vi "Clear Controls.vi"(8 "error in (no error)":errorcluster, 10 "Array 2":refnum<vi>[](array[refnum]), 11 "Array":refnum<vi>[](array[refnum])) -> (0 "error out":errorcluster)   [LabVIEW 2020]
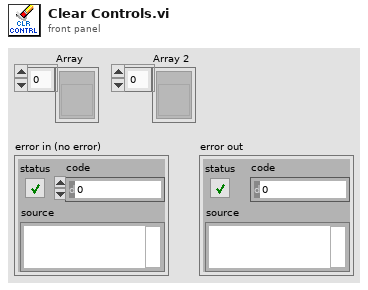
[diagram p1: front panel]
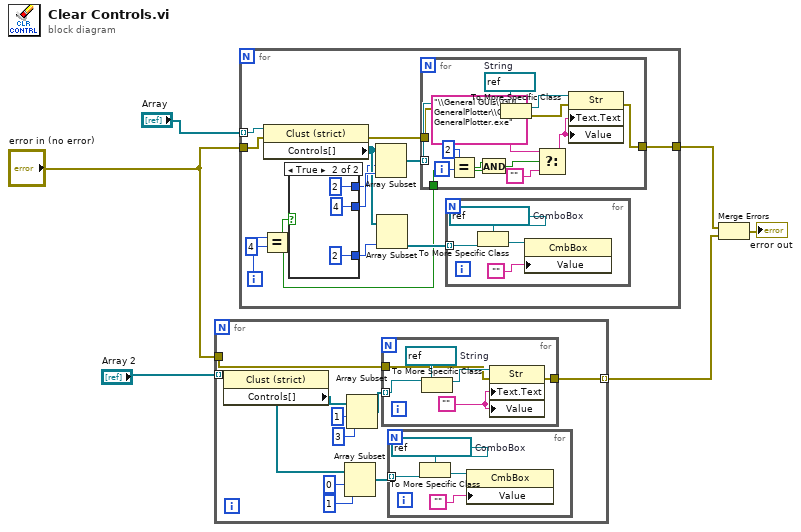
[diagram p0: block diagram]
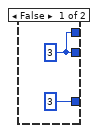
[diagram p2: hidden frame]
diagram:
  n1 = for {
    tunnel: "Array 2" -> [w13] mode=indexing
    tunnel: "error in (no error)" -> [w12]
    tunnel: [w7] -> w3 mode=indexing
    n2 = property class="Clust (strict)"(reference=w13) -> ("Controls[]"=w11:refnum<vi>[])  [unwired: 1 in, 2 out]
    n3 = Array Subset(array=w11, index=0, length=1) -> (w8:refnum<vi>[])
    n4 = Array Subset(array=w11, index=1, length=3) -> (w16:refnum<vi>[])
    n5 = for {
      tunnel: w16 -> [w26] mode=indexing
      tunnel: [w22] -> w7
      tunnel: w12 -> [w21]
      w23 = ""
      w25 = refnum<vi> refnum  # String
      n6 = To More Specific Class(target class=w25, reference=w26) -> (specific class reference=w24:refnum<vi>)  [unwired: 1 in, 1 out]
      n7 = property class="Str"(reference=w24, error in=w21, "Text.Text"=w23, "Value"=w23) -> (error out=w22:errorcluster)  [unwired: 1 out]
    }
    n8 = for {
      tunnel: w8 -> [w20] mode=indexing
      w19 = refnum<vi> refnum  # ComboBox
      n9 = To More Specific Class(target class=w19, reference=w20) -> (specific class reference=w18:refnum<vi>)  [unwired: 1 in, 1 out]
      n10 = property class="CmbBox"(reference=w18, "Value"="") -> ()  [unwired: 1 in, 2 out]
    }
  }
  n11 = for {
    tunnel: "Array" -> [w39] mode=indexing
    tunnel: "error in (no error)" -> [w30]
    tunnel: [w28] -> w4
    i -> [w33]
    n12 = Equal?(x=w33, y=4 ("length")) -> (x = y?=w27:bool)
    n13 = property class="Clust (strict)"(reference=w39, error in=w30) -> (error out=w29:errorcluster, "Controls[]"=w36:refnum<vi>[])  [unwired: 1 out]
    n14 = case shown="True" w27 {
      tunnel: [w58 4 ("length")] -> w38
      tunnel: [3 ("length") 2 ("length")] -> w35
      tunnel: [w58 2 ("length")] -> w31
      frame False {
        w58 = 3 ("length")
      }
      frame True {
      }
    }
    n15 = Array Subset(array=w36, index=w31, length=w38) -> (w37:refnum<vi>[])
    n16 = Array Subset(array=w36, length=w35) -> (w34:refnum<vi>[])  [unwired: 1 in]
    n17 = for {
      tunnel: w37 -> [w57] mode=indexing
      tunnel: w29 -> [w54]
      tunnel: [w52] -> w28
      tunnel: w27 -> [w45]
      i -> [w51]
      w56 = refnum<vi> refnum  # String
      n18 = Equal?(x=2, y=w51) -> (x = y?=w46:bool)
      n19 = And(x=w46, y=w45) -> (x .and. y?=w44:bool)
      n20 = To More Specific Class(target class=w56, reference=w57, error in=w54) -> (specific class reference=w55:refnum<vi>, error out=w53:errorcluster)
      n21 = Select(t="\\General GUIs\\GUI_GeneralPlotter\\GUI_GeneralPlotter.exe", s=w44, f="") -> (s? t:f=w49:string)
      n22 = property class="Str"(reference=w55, error in=w53, "Text.Text"=w49, "Value"=w49) -> (error out=w52:errorcluster)  [unwired: 1 out]
    }
    n23 = for {
      tunnel: w34 -> [w43] mode=indexing
      w42 = refnum<vi> refnum  # ComboBox
      n24 = To More Specific Class(target class=w42, reference=w43) -> (specific class reference=w41:refnum<vi>)  [unwired: 1 in, 1 out]
      n25 = property class="CmbBox"(reference=w41, "Value"="") -> ()  [unwired: 1 in, 2 out]
    }
  }
  n26 = Merge Errors(w4, w3) -> (→"error out":errorcluster)
